vi "TemperatureSensors_READ.vi"(8 "Error IN":errorcluster, 9 "CS Configuration":T1={"CS Channel"=10, "CS Logic Level"=enum."Active Low"}, 11 "LINX Resource IN":T3) -> (0 "Error OUT":errorcluster, 1 "CJC Temperature [°C]":dbl, 2 "Temperature [°C]":dbl format="%3.2f", 3 "LINX Resource OUT":T3, 4 "Error Array":bool[](array[boolean])=[FALSE, FALSE, FALSE, FALSE, TRUE, FALSE, TRUE, TRUE], 5 "STOP Condition":bool)   [LabVIEW 2017]
doc: "This VI is used to read values from Sensortechnics pressure transducers (HMI-Series) via the I²C- Bus Protocoll."
uses:
  <vilib>/MakerHub/LINX/Private/Type Defs/LINX Ref.ctl
  <vilib>/MakerHub/LINX/Private/Type Defs/Platform.ctl
  <vilib>/MakerHub/LINX/Private/Type Defs/Interface.ctl
  <vilib>/MakerHub/LINX/Private/Device/Type Defs/LINX Device Config.ctl
  <vilib>/MakerHub/LINX/Private/Device/Type Defs/TCP Config.ctl
  <vilib>/MakerHub/LINX/Private/Device/Type Defs/Channels.ctl
  <vilib>/MakerHub/LINX/Public/Peripherals/SPI/SPI CS Config.ctl
  <vilib>/MakerHub/LINX/Private/Type Defs/Peripherals/SPI/SPI CS Logic Level.ctl
  <vilib>/MakerHub/LINX/Public/Peripherals/SPI/SPI Write Read N Frames.vi
  <vilib>/MakerHub/LINX/Private/Local IO/LinxSpiWriteRead.vi
  <vilib>/MakerHub/LINX/Public/Utilities/Check Channel.vi
  <vilib>/MakerHub/LINX/Private/Utilties/Generate Error.vi
  <vilib>/MakerHub/LINX/LMH-LINX.lvlib
  <vilib>/MakerHub/LINX/Private/Device/Device.lvlib
panel:
  out "Read Data":u8[](array[numeric])
  # "OUTPUT"
  # "INPUT"
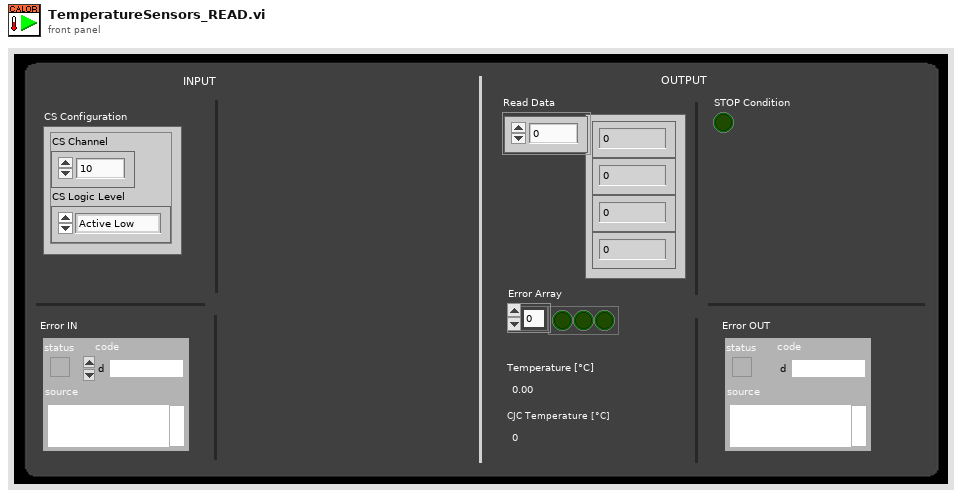
[diagram p1: front panel]
types:
  T1 = typedef "LMH-LINX.lvlib/SPI CS Config.ctl" = cluster{"CS Channel":u8, "CS Logic Level":T2}
  T2 = typedef "LMH-LINX.lvlib/SPI CS Logic Level.ctl" = enum8{"Active Low", "Active High"}
  T3 = typedef "LMH-LINX.lvlib/LINX Ref.ctl" = cluster{"IO":T4, "Interface":T5, "LINX Device Config":T6}
  T4 = typedef "LMH-LINX.lvlib/Platform.ctl" = enum16{"Remote", "Local"}
  T5 = typedef "LMH-LINX.lvlib/Interface.ctl" = enum16{"Serial", "TCP"}
  T6 = typedef "LMH-LINX.lvlib/Device.lvlib/LINX Device Config.ctl" = cluster{"Interface":T5, "COM Port":refnum<visa-resource-name>, "TCP Configuration":T7, "Device Family":u8, "Device ID":u8, "Device Name":string, "TCP Ref":refnum<k5>, "Channels":T8}
  T7 = typedef "LMH-LINX.lvlib/Device.lvlib/TCP Config.ctl" = cluster{"IP Address":string, "Port":u16}
  T8 = typedef "LMH-LINX.lvlib/Channels.ctl" = cluster{"DI":u8[], "DO":u8[], "AI":u8[], "AO":u8[], "PWM":u8[], "QE":u8[], "UART":u8[], "I2C 2":u8[], "SPI":u8[], "CAN":u8[], "Servo":u8[], "AI Ref (V)":dbl, "AI Resolution (Bits)":u8, "AO Ref (V)":dbl, "AO Resolution (Bits)":u8}
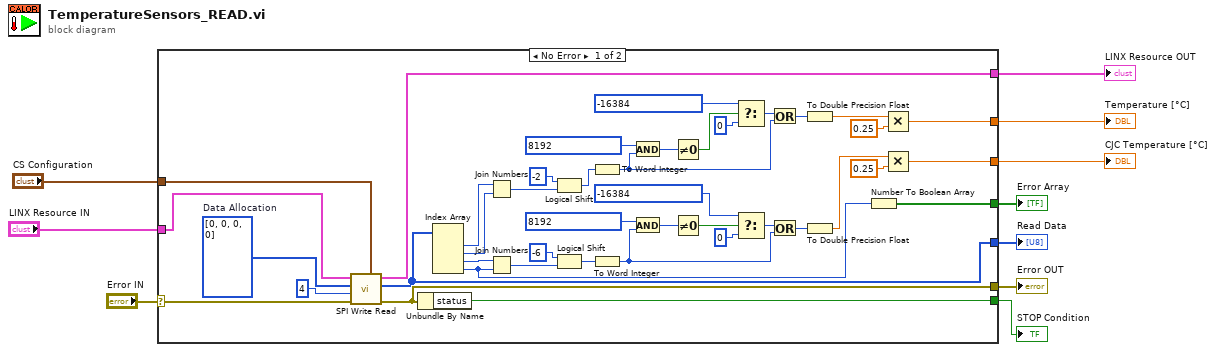
[diagram p0: block diagram]
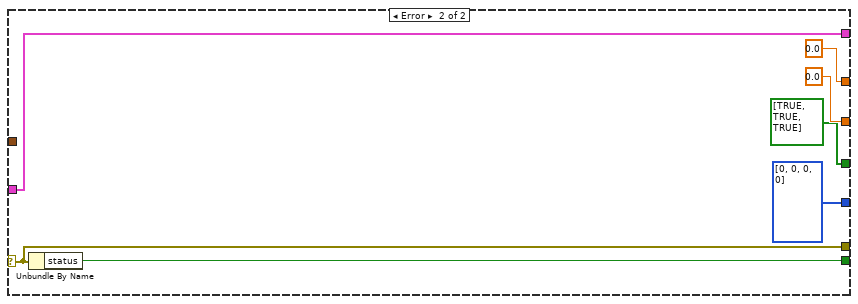
[diagram p2: hidden frame]
diagram:
  n1 = case shown="No Error" "Error IN" {
    selector: "Error IN" -> [w48 w57]
    tunnel: [w52 w59] -> w10
    tunnel: [w51 w57] -> w9
    tunnel: "LINX Resource IN" -> [w50 w58]
    tunnel: [w49 w58] -> w7
    tunnel: "CS Configuration" -> [w47 _]
    tunnel: [w13 0.0 ("number: 0 to 1")] -> w4
    tunnel: [w14 0.0 ("number: 0 to 1")] -> w3
    tunnel: [w12 bool[] [TRUE, TRUE, TRUE] ("Boolean array")] -> w2
    tunnel: [w11 u8[] [0, 0, 0, 0] ("Read Data")] -> w1
    frame No Error {
      w45 = u8[] [0, 0, 0, 0]  # Data Allocation
      n2 = call-poly <vilib>:"SPI Write Read.vi"("CS Configuration"=w47, "Error In"=w48, "SPI Frame Size"=u8 4 ("SPI Frame Size (0)"), "Data"=w45, "LINX Resource"=w50) -> ("Error Out"=w51:errorcluster, "Read Data"=w11:u8[], "LINX Resource"=w49:T3)  [unwired: 4 in]
      n3 = Unbundle By Name(w51) -> ("status"=w52:bool)
      n4 = Index Array(array=w11) -> (element #1=w19:u8, element #2=w18:u8, element #3=w17:u8, element #4=w16:u8)  [unwired: 4 in]
      n5 = Join Numbers(hi=w19, lo=w18) -> ((hi.lo)=w43:u16)
      n6 = Join Numbers(hi=w17, lo=w16) -> ((hi.lo)=w21:u16)
      n7 = Logical Shift(y=i16 -2, x=w43) -> (x << y=w36:u16)
      n8 = Logical Shift(y=i8 -6, x=w21) -> (x << y=w25:u16)
      n9 = To Word Integer(number=w36) -> (16bit integer=w34:i16)
      n10 = To Word Integer(number=w25) -> (16bit integer=w23:i16)
      n11 = And(x=i16 8192, y=w34) -> (x .and. y?=w40:i16)
      n12 = And(x=i16 8192, y=w23) -> (x .and. y?=w29:i16)
      n13 = Not Equal To 0?(x=w40) -> (x != 0?=w42:bool)
      n14 = Not Equal To 0?(x=w29) -> (x != 0?=w32:bool)
      n15 = Select(t=i16 -16384, s=w42, f=i16 0) -> (s? t:f=w35:i16)
      n16 = Select(t=i16 -16384, s=w32, f=i16 0) -> (s? t:f=w24:i16)
      n17 = Or(x=w35, y=w34) -> (x .or. y?=w33:i16)
      n18 = Or(x=w24, y=w23) -> (x .or. y?=w22:i16)
      n19 = To Double Precision Float(number=w33) -> (double precision float=w38:dbl)
      n20 = To Double Precision Float(number=w22) -> (double precision float=w27:dbl)
      n21 = Number To Boolean Array(number=w16) -> (Boolean array=w12:bool[])
      n22 = Multiply(x=w38, y=0.25) -> (x*y=w13:dbl)
      n23 = Multiply(x=w27, y=0.25) -> (x*y=w14:dbl)
    }
    frame Error {
      n24 = Unbundle By Name(w57) -> ("status"=w59:bool)
    }
  }
  "Error OUT" <- w9
  "STOP Condition" <- w10
  "LINX Resource OUT" <- w7
  "Temperature [°C]" <- w4
  "CJC Temperature [°C]" <- w3
  "Error Array" <- w2
  "Read Data" <- w1
